vi "Stop PVProxy.vi"(8 "Error In":errorcluster, 11 "CS++BaseActor in":refnum<class "CS++BaseActor.lvclass">) -> (0 "Error Out":errorcluster, 3 "CS++BaseActor out":refnum<class "CS++BaseActor.lvclass">)   [LabVIEW 2016, in "CS++BaseActor.lvlib" / "CS++BaseActor.lvclass"]
doc: "Stop PVProxy."
uses:
  CS++BaseActor.lvclass
  CS++BaseActor.lvclass/CS++BaseActor.ctl
  <vilib>/ActorFramework/Message Enqueuer/Message Enqueuer.lvclass/Message Enqueuer.ctl
  <vilib>/ActorFramework/Message Enqueuer/Enqueue.vi
  <vilib>/ActorFramework/Stop Msg/Stop Msg.lvclass
  C:/Program Files (x86)/National Instruments/LabVIEW 2016/vi.lib/ActorFramework/Message/Message.lvclass
  <vilib>/ActorFramework/Message Priority Queue/Priority Enqueue.vi
  <vilib>/ActorFramework/Message Enqueuer/Message Enqueuer.lvclass
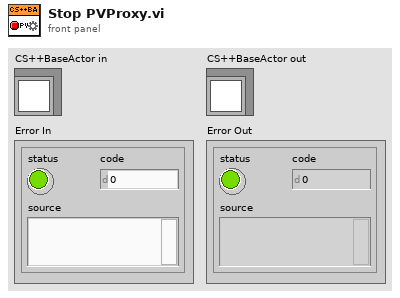
[diagram p1: front panel]
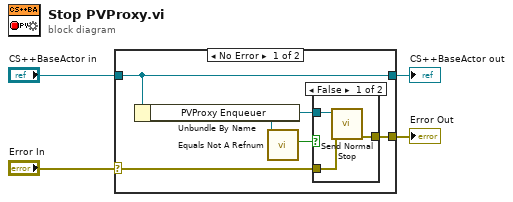
[diagram p0: block diagram]
diagram:
  n1 = case shown="No Error" "Error In" {
    selector: "Error In" -> [w7 w15]
    tunnel: [w6 w15] -> w3
    tunnel: [w9 w14] -> w1
    tunnel: "CS++BaseActor in" -> [w9 w14]
    frame No Error {
      n2 = Unbundle By Name(w9) -> ("PVProxy Enqueuer"=w8:refnum<class "Message Enqueuer.lvclass">)
      n3 = call <vilib>:"Equals Not A Refnum.vi"("Message Enqueuer"=w8) -> ("Not a refnum?"=w5:bool)  [unwired: 10 in]
      n4 = case shown="False" w5 {
        tunnel: w8 -> [w12 _]
        tunnel: w7 -> [w11 w13]
        tunnel: [w10 w13] -> w6
        frame False {
          n5 = call <vilib>:"Send Normal Stop.vi"("error in (no error)"=w11, "Message Enqueuer"=w12) -> ("error out"=w10:errorcluster)  [unwired: 9 in]
        }
        frame True {
        }
      }
    }
    frame Error {
    }
  }
  "Error Out" <- w3
  "CS++BaseActor out" <- w1
